vi "TL read IR sensors.vi"(1 "GPS":cluster{"X pos":i32, "Y pos":i32, "Heading":dbl}, 2 "IR Sensors":T1(array[cluster]), 3 "Pool image\nPixels (U32)":u32[][](array[numeric])) -> (0 "IR Sensors out":T1(array[cluster]))   [LabVIEW 2014]
panel:
  out "boat color":u32
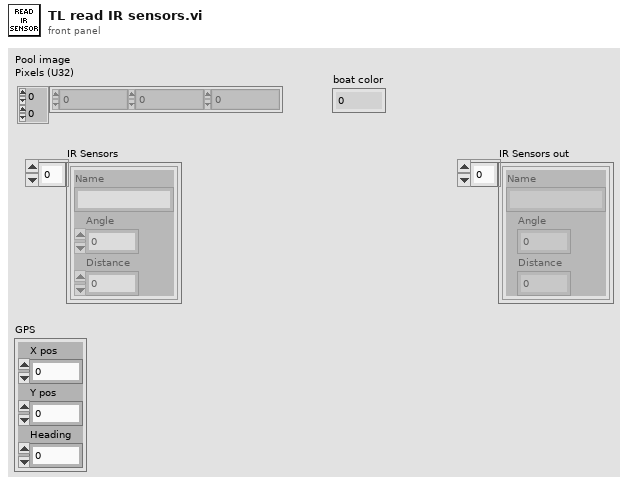
[diagram p1: front panel]
types:
  T1 = cluster{"Name":string, "Angle":dbl, "Distance":dbl}[]
  T2 = cluster{"Name":string, "Angle":dbl, "Distance":dbl}
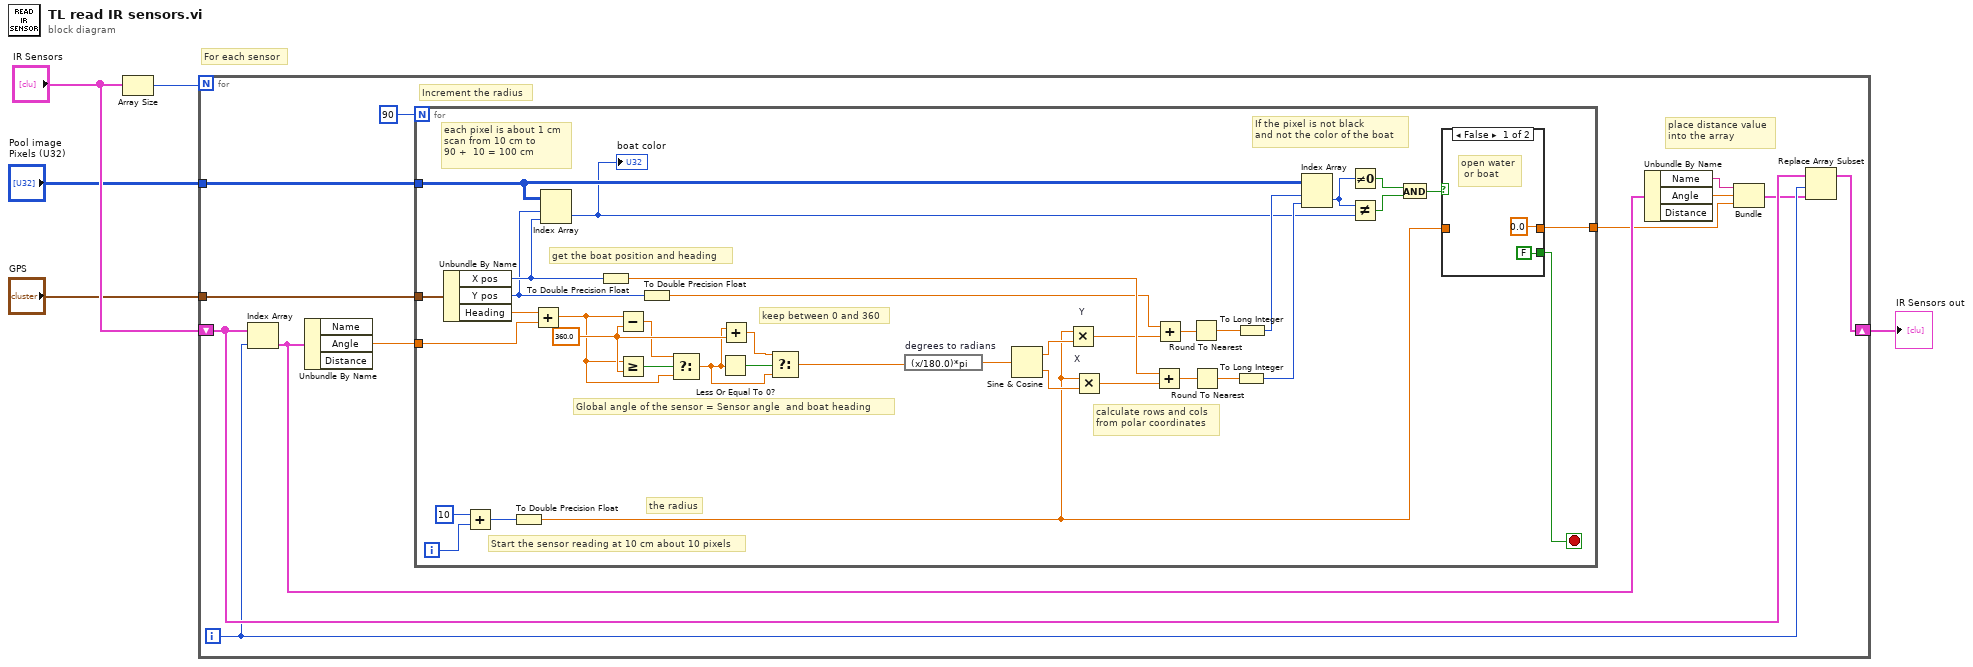
[diagram p0: block diagram]
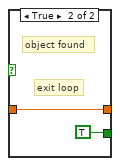
[diagram p2: hidden frame]
diagram:
  # "For each sensor"
  n1 = Array Size(array="IR Sensors") -> (size(s)=w5:i32)
  n2 = for {
    N: w5 -> [_]
    shift-right: [w6] -> w1
    shift-left: "IR Sensors" -> [w13]
    tunnel: "GPS" -> [w16]
    tunnel: "Pool image\nPixels (U32)" -> [w14]
    i -> [w12]
    # "place distance value\ninto the array"
    # "Increment the radius"
    n3 = Index Array(array=w13, index=w12) -> (element=w11:T2)
    n4 = Unbundle By Name(w11) -> ("Angle"=w15:dbl)  [unwired: 2 out]
    n5 = for {
      N: 90 -> [_]
      tunnel: w16 -> [w53]
      tunnel: w15 -> [w51]
      tunnel: w14 -> [w28]
      tunnel: [w20] -> w8
      i -> [w42]
      stop <- w21 stop-if-true
      w49 = 360.0
      # "If the pixel is not black \nand not the color of the boat"
      # "keep between 0 and 360"
      # "each pixel is about 1 cm\nscan from 10 cm to \n90 +  10 = 100 cm"
      # "Start the sensor reading at 10 cm about 10 pixels"
      # "Global angle of the sensor = Sensor angle  and boat heading"
      # "the radius"
      # "get the boat position and heading"
      # "calculate rows and cols\nfrom polar coordinates"
      n6 = Unbundle By Name(w53) -> ("X pos"=w40:i32, "Y pos"=w38:i32, "Heading"=w52:dbl)
      n7 = Add(x=10, y=w42) -> (x+y=w43:i32)
      n8 = To Double Precision Float(number=w43) -> (double precision float=w22:dbl)
      n9 = Add(x=w52, y=w51) -> (x+y=w45:dbl)
      n10 = Index Array(array=w28, index (row)=w38, index (col)=w40) -> (element=w26:u32)
      "boat color" <- w26
      n11 = To Double Precision Float(number=w40) -> (double precision float=w39:dbl)
      n12 = Subtract(x=w45, y=w49) -> (x-y=w47:dbl)
      n13 = Greater Or Equal?(x=w45, y=w49) -> (x >= y?=w46:bool)
      n14 = To Double Precision Float(number=w38) -> (double precision float=w37:dbl)
      n15 = Select(t=w47, s=w46, f=w45) -> (s? t:f=w19:dbl)
      n16 = Less Or Equal To 0?(x=w19) -> (x <= 0?=w48:bool)
      n17 = Add(x=w19, y=w49) -> (x+y=w50:dbl)
      n18 = Select(t=w50, s=w48, f=w19) -> (s? t:f=w18:dbl)
      n19 = expression code="(x/180.0)*pi" "degrees to radians"(w18) -> (w44:dbl)
      n20 = Sine & Cosine(0:w44) -> (1:w54:dbl, 2:w55:dbl)
      n21 = Multiply "Y"(x=w22, y=w54) -> (x*y=w36:dbl)
      n22 = Multiply "X"(x=w22, y=w55) -> (x*y=w35:dbl)
      n23 = Add(x=w39, y=w35) -> (x+y=w33:dbl)
      n24 = Add(x=w37, y=w36) -> (x+y=w34:dbl)
      n25 = Round To Nearest(number=w34) -> (nearest integer value=w31:dbl)
      n26 = Round To Nearest(number=w33) -> (nearest integer value=w32:dbl)
      n27 = To Long Integer(number=w32) -> (32bit integer=w30:i32)
      n28 = To Long Integer(number=w31) -> (32bit integer=w29:i32)
      n29 = Index Array(array=w28, index (row)=w29, index (col)=w30) -> (element=w27:u32)
      n30 = Not Equal To 0?(x=w27) -> (x != 0?=w24:bool)
      n31 = Not Equal?(x=w27, y=w26) -> (x != y?=w25:bool)
      n32 = And(x=w24, y=w25) -> (x .and. y?=w23:bool)
      n33 = case shown="False" w23 {
        tunnel: w22 -> [_ w58]
        tunnel: [FALSE TRUE] -> w21
        tunnel: [0.0 w58] -> w20
        frame False {
          # "open water\n or boat"
        }
        frame True {
          # "exit loop"
          # "object found"
        }
      }
    }
    n34 = Unbundle By Name(w11) -> ("Name"=w10:string, "Angle"=w9:dbl)  [unwired: 1 out]
    n35 = Bundle("Name"=w10, "Angle"=w9, w8) -> (w7:cluster{"Name":string, "Angle":dbl, dbl})  [unwired: 1 in]
    n36 = Replace Array Subset(array=w13, new element=w7, index=w12) -> (w6:T1)
  }
  "IR Sensors out" <- w1
